vi "PicoScope5000aGetTriggerInfo.vi"(0 "handle in":i16, 5 "Rapid Block Acquisition Settings":T2={"fromSegmentIndex"=0, "toSegmentIndex"=1000} {"toSegmentIndex" format="%.4p"; "fromSegmentIndex" format="%.4p"}, 9 "Sample Rate":sgl, 11 "error in":errorcluster) -> (4 "handle out":i16, 6 "Trigger Info":T1(array[cluster]), 10 "Trigger Offsets":cluster{u64, sgl}[](array[cluster]) {"?" format="%#_5p"}, 15 "error out":errorcluster)   [LabVIEW 2020]
doc: "This VI gets a set of blocks captured using rapid block mode. It outputs two-dimensional arrays for each channel that contain data from all the requested captures."
uses:
  Segment Range.ctl
  ps5000a.dll
panel:
  out "Number of Captures":u32=1
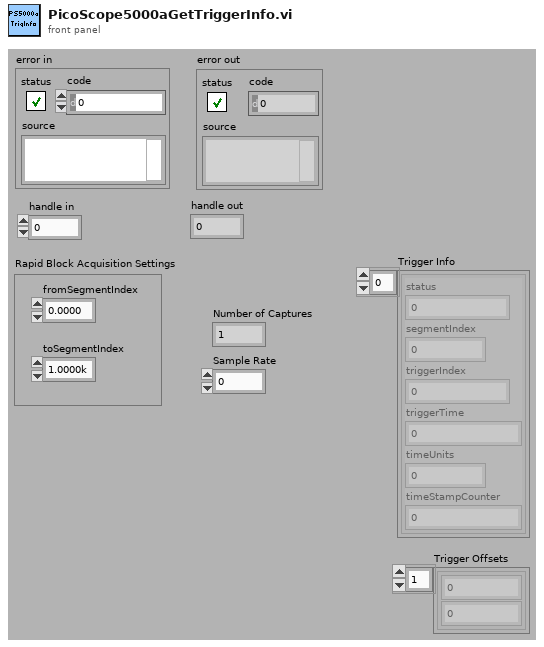
[diagram p1: front panel]
types:
  T1 = cluster{"status":u32, "segmentIndex":u32, "triggerIndex":u32, "triggerTime":i64, "timeUnits":i16, "timeStampCounter":u64}[]
  T2 = typedef "Segment Range.ctl" = cluster{"fromSegmentIndex":u64, "toSegmentIndex":u64}
  T3 = cluster{"status":u32, "segmentIndex":u32, "triggerIndex":u32, "triggerTime":i64, "timeUnits":i16, "reserved0":i16, "timeStampCounter":u64}
  T4 = cluster{"status":u32, "segmentIndex":u32, "triggerIndex":u32, "triggerTime":i64, "timeUnits":i16, "timeStampCounter":u64}
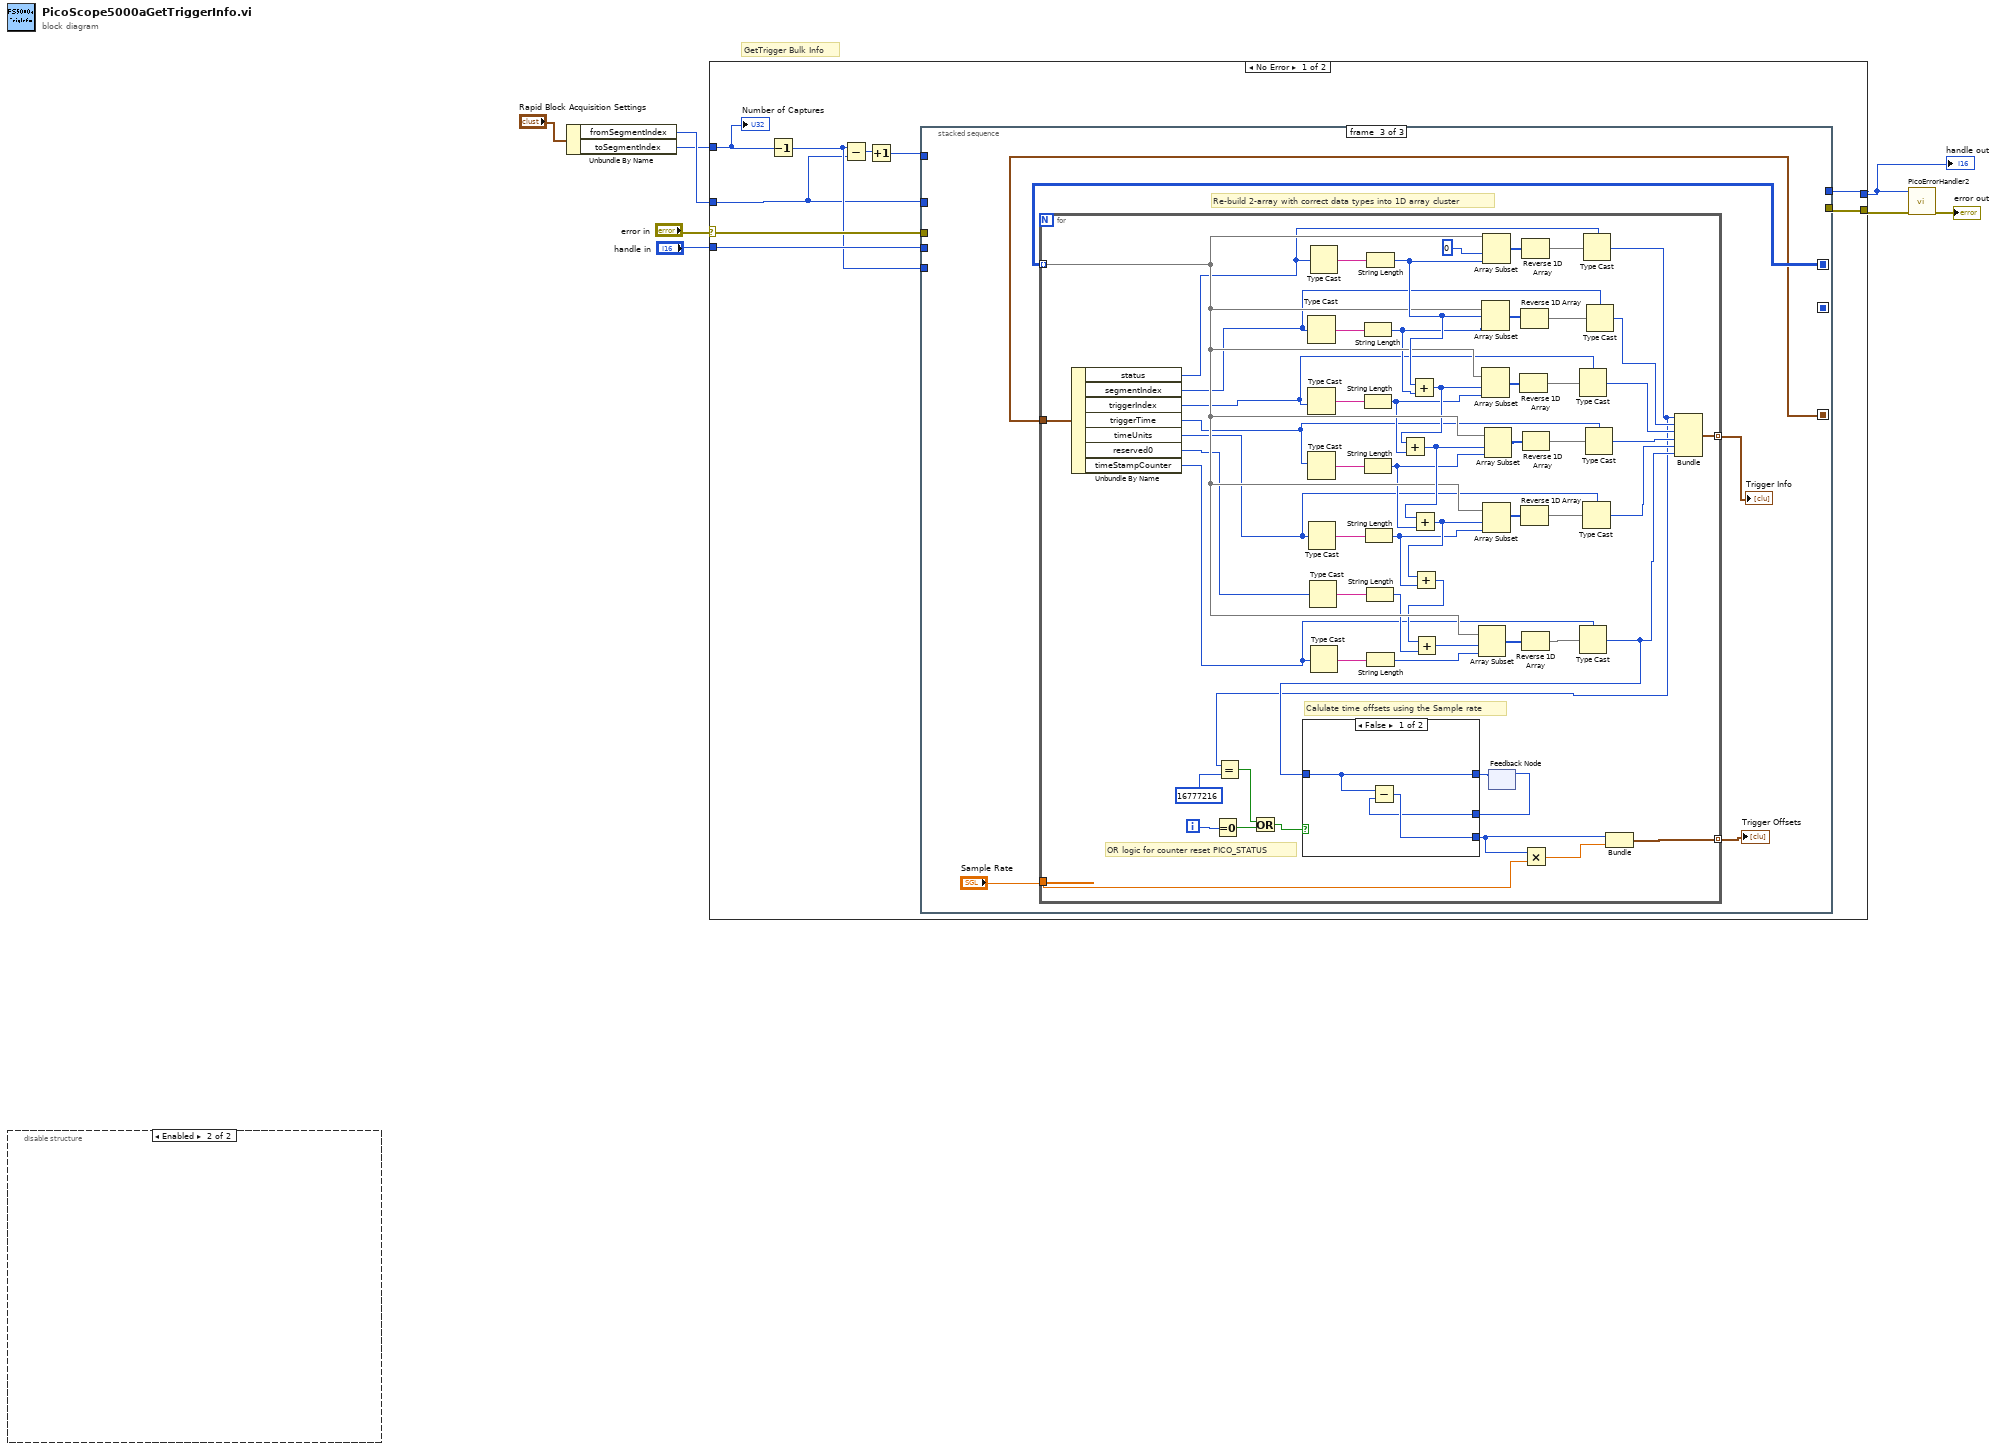
[diagram p0: block diagram]
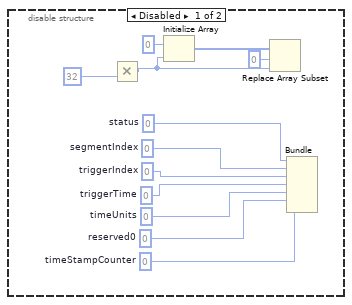
[diagram p2: hidden frame]
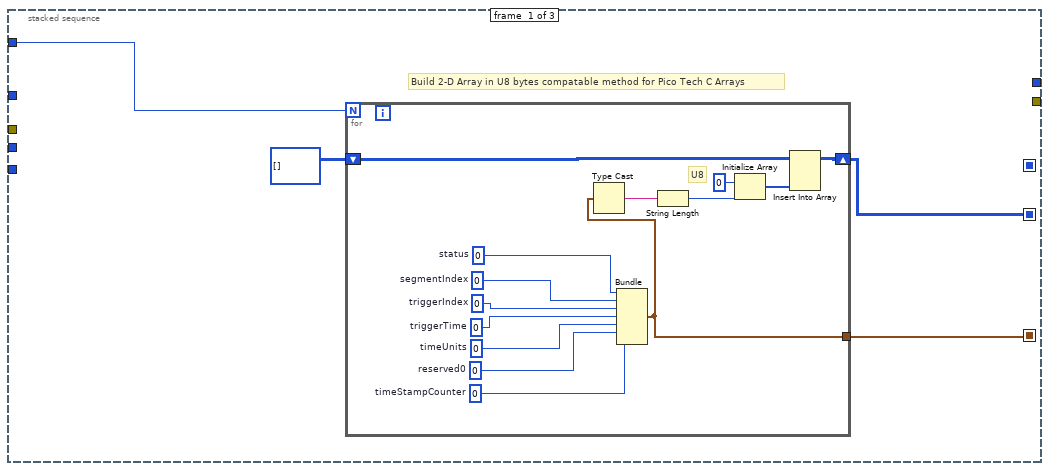
[diagram p3: hidden frame]
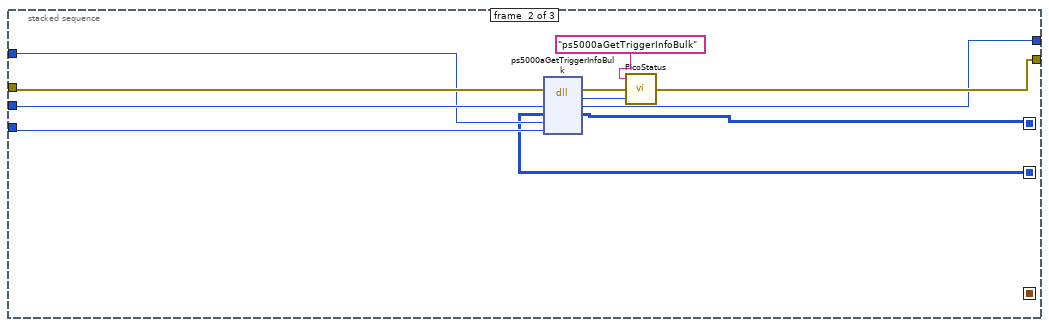
[diagram p4: hidden frame]
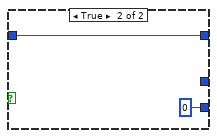
[diagram p5: hidden frame]
diagram:
  # "GetTrigger Bulk Info"
  n1 = disable-structure shown="Enabled" {
    frame Disabled {
      w16 = u64 0  # timeStampCounter
      w14 = i16 0  # reserved0
      w15 = i16 0  # timeUnits
      w17 = i64 0  # triggerTime
      w18 = u32 0  # triggerIndex
      w19 = u32 0  # segmentIndex
      w20 = u32 0  # status
      n2 = Multiply(y=u32 32) -> (x*y=w12:u32)  [unwired: 1 in]
      n3 = Initialize Array(u8 0 ("element"), w12) -> (w13:u8[])
      n4 = Replace Array Subset(array=w13, new element=w12, index=0) -> ()  [unwired: 1 out]
      n5 = Bundle("status"=w20, "segmentIndex"=w19, "triggerIndex"=w18, "triggerTime"=w17, "timeUnits"=w15, "reserved0"=w14, "timeStampCounter"=w16) -> ()  [unwired: 1 in, 1 out]
    }
    frame Enabled {
    }
  }
  n6 = Unbundle By Name("Rapid Block Acquisition Settings") -> ("fromSegmentIndex"=w2:u64, "toSegmentIndex"=w1:u64)
  n7 = case shown="No Error" "error in" {
    selector: "error in" -> [w28 w130]
    tunnel: [w25 w130] -> w5
    tunnel: "handle in" -> [w27 w129]
    tunnel: [w24 w129] -> w6
    tunnel: w1 -> [w29 _]
    tunnel: w2 -> [w21 _]
    frame No Error {
      n8 = Decrement(x=w29) -> (x-1=w26:u64)
      n9 = Subtract(x=w26, y=w21) -> (x-y=w23:u64)
      n10 = Increment(x=w23) -> (x+1=w22:u64)
      n11 = stacked-sequence {
        seq-local: [w31 _ _] -> [_ w51 _]
        seq-local: [w30 _ _] -> [_ w49 _]
        seq-local: [_ w50 _] -> [_ _ w64]
        seq-local: [_ w49 _] -> [_ _ w60]
        tunnel: w22 -> [w33 _ _]
        tunnel: w28 -> [_ w56 _]
        tunnel: w27 -> [_ w54 _]
        tunnel: w21 -> [_ w53 _]
        tunnel: w26 -> [_ w52 _]
        tunnel: [_ w55 _] -> w25
        tunnel: [_ w48 _] -> w24
        frame #0 {
          # "Build 2-D Array in U8 bytes compatable method for Pico Tech C Arrays"
          n12 = for {
            N: w33 -> [_]
            shift-right: [w35] -> w31
            shift-left: u8[][] [] -> [w36]
            tunnel: [w34] -> w30
            w43 = u64 0  # timeStampCounter
            w41 = i16 0  # reserved0
            w42 = i16 0  # timeUnits
            w44 = i64 0  # triggerTime
            w45 = u32 0  # triggerIndex
            w46 = u32 0  # segmentIndex
            w47 = u32 0  # status
            # "U8"
            n13 = Bundle("status"=w47, "segmentIndex"=w46, "triggerIndex"=w45, "triggerTime"=w44, "timeUnits"=w42, "reserved0"=w41, "timeStampCounter"=w43) -> (w34:T3)  [unwired: 1 in]
            n14 = Type Cast(x=w34) -> (*(type *) &x=w40:string)  [unwired: 1 in]
            n15 = String Length(string=w40) -> (length=w38:i32)
            n16 = Initialize Array(u8 0 ("element"), w38) -> (w37:u8[])
            n17 = Insert Into Array(array=w36, new element=w37) -> (w35:u8[][])  [unwired: 2 in]
          }
        }
        frame #1 {
          n18 = dll-call lib="ps5000a.dll" fn="ps5000aGetTriggerInfoBulk" ("ps3000.dll:_ps3000_open_unit@0")(error in=w56, "handle"=w54, "triggerInfo"=w51, "fromSegmentIndex"=w53, "toSegmentIndex"=w52) -> (error out=w59:errorcluster, "PICO_STATUS"=w58:u32, "handle"=w48:i16, "triggerInfo"=w50:u8[][])  [unwired: 4 in, 1 out]
          n19 = call "PicoStatus.vi"("PICO STATUS"=w58, "error in"=w59, "source"="ps5000aGetTriggerInfoBulk") -> ("error out"=w55:errorcluster)
        }
        frame #2 {
          # "Re-build 2-array with correct data types into 1D array cluster"
          n20 = for {
            tunnel: w64 -> [w85] mode=indexing
            tunnel: [w120] -> w63 mode=indexing
            tunnel: [w103] -> w62 mode=indexing
            tunnel: "Sample Rate" -> [w102]
            tunnel: w60 -> [w72]
            i -> [w106]
            # "Calulate time offsets using the Sample rate"
            # "OR logic for counter reset PICO_STATUS"
            n21 = Unbundle By Name(w72) -> ("status"=w71:u32, "segmentIndex"=w70:u32, "triggerIndex"=w65:u32, "triggerTime"=w66:i64, "timeUnits"=w67:i16, "reserved0"=w68:i16, "timeStampCounter"=w69:u64)
            n22 = Equal To 0?(x=w106) -> (x = 0?=w77:bool)
            n23 = Type Cast(x=w70) -> (*(type *) &x=w98:string)  [unwired: 1 in]
            n24 = Type Cast(x=w65) -> (*(type *) &x=w97:string)  [unwired: 1 in]
            n25 = Type Cast(x=w66) -> (*(type *) &x=w96:string)  [unwired: 1 in]
            n26 = Type Cast(x=w67) -> (*(type *) &x=w95:string)  [unwired: 1 in]
            n27 = Type Cast(x=w68) -> (*(type *) &x=w94:string)  [unwired: 1 in]
            n28 = Type Cast(x=w71) -> (*(type *) &x=w99:string)  [unwired: 1 in]
            n29 = Type Cast(x=w69) -> (*(type *) &x=w89:string)  [unwired: 1 in]
            n30 = String Length(string=w98) -> (length=w83:i32)
            n31 = String Length(string=w97) -> (length=w81:i32)
            n32 = String Length(string=w96) -> (length=w80:i32)
            n33 = String Length(string=w95) -> (length=w79:i32)
            n34 = String Length(string=w94) -> (length=w78:i32)
            n35 = String Length(string=w99) -> (length=w90:i32)
            n36 = String Length(string=w89) -> (length=w87:i32)
            n37 = Add(x=w90, y=w83) -> (x+y=w82:i32)
            n38 = Add(x=w82, y=w81) -> (x+y=w93:i32)
            n39 = Add(x=w93, y=w80) -> (x+y=w92:i32)
            n40 = Add(x=w92, y=w79) -> (x+y=w84:i32)
            n41 = Add(x=w84, y=w78) -> (x+y=w88:i32)
            n42 = Array Subset(array=w85, index=w88, length=w87) -> (w86:u8[])
            n43 = Array Subset(array=w85, index=w90, length=w83) -> (w119:u8[])
            n44 = Array Subset(array=w85, index=w82, length=w81) -> (w114:u8[])
            n45 = Array Subset(array=w85, index=0, length=w90) -> (w117:u8[])
            n46 = Array Subset(array=w85, index=w92, length=w79) -> (w111:u8[])
            n47 = Array Subset(array=w85, index=w93, length=w80) -> (w113:u8[])
            n48 = feedback #1() -> (w104:u64)  [unwired: 1 in]
            n49 = Reverse 1D Array(array=w114) -> (reversed array=w115:u8[])
            n50 = Reverse 1D Array(array=w119) -> (reversed array=w118:u8[])
            n51 = Reverse 1D Array(array=w111) -> (reversed array=w110:u8[])
            n52 = Reverse 1D Array(array=w117) -> (reversed array=w116:u8[])
            n53 = Reverse 1D Array(array=w86) -> (reversed array=w109:u8[])
            n54 = Reverse 1D Array(array=w113) -> (reversed array=w112:u8[])
            n55 = Type Cast(type=w65, x=w115) -> (*(type *) &x=w123:u32)
            n56 = Type Cast(type=w69, x=w109) -> (*(type *) &x=w107:u64)
            n57 = Type Cast(type=w67, x=w110) -> (*(type *) &x=w121:i16)
            n58 = Type Cast(type=w71, x=w116) -> (*(type *) &x=w73:u32)
            n59 = Equal?(x=w73, y=u32 16777216 ("status")) -> (x = y?=w75:bool)
            n60 = Or(x=w75, y=w77) -> (x .or. y?=w76:bool)
            n61 = case shown="False" w76 {
              tunnel: w107 -> [w125 w128]
              tunnel: [w125 w128] -> w105
              tunnel: w104 -> [w124 _]
              tunnel: [w126 u64 0] -> w101
              frame False {
                n62 = Subtract(x=w125, y=w124) -> (x-y=w126:u64)
              }
              frame True {
              }
            }
            n63 = feedback-in #1(w105) -> ()
            n64 = Multiply(x=w101, y=w102) -> (x*y=w100:sgl)
            n65 = Type Cast(type=w66, x=w112) -> (*(type *) &x=w122:i64)
            n66 = Type Cast(type=w70, x=w118) -> (*(type *) &x=w108:u32)
            n67 = Bundle(w101, w100) -> (w103:cluster{u64, sgl})  [unwired: 1 in]
            n68 = Bundle("status"=w73, "segmentIndex"=w108, "triggerIndex"=w123, "triggerTime"=w122, "timeUnits"=w121, "timeStampCounter"=w107) -> (w120:T4)  [unwired: 1 in]
          }
          "Trigger Info" <- w63
          "Trigger Offsets" <- w62
        }
      }
      "Number of Captures" <- w29
    }
    frame Error {
    }
  }
  "handle out" <- w6
  n69 = call "PicoErrorHandler2.vi"("error in (no error)"=w5, "handle In"=w6) -> ("error out"=→"error out":errorcluster)  [unwired: 9 in]
